vi "Read Needs rebuilding.vi"(11 "ProjectItem in":refnum<class "ProjectItem.lvclass">) -> (2 "Needs rebuilding":bool, 3 "ProjectItem out":refnum<class "ProjectItem.lvclass">)   [LabVIEW 2019, in "SolutionBuilder.lvlib" / "ProjectItem.lvclass"]
uses:
  ProjectItem.lvclass
  ProjectItem.lvclass/ProjectItem.ctl
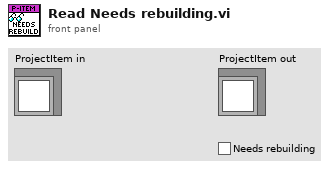
[diagram p1: front panel]
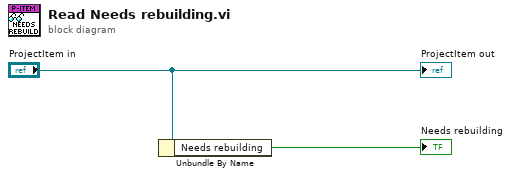
[diagram p0: block diagram]
diagram:
  n1 = Unbundle By Name("ProjectItem in") -> ("Needs rebuilding"=→"Needs rebuilding":bool)
  "ProjectItem out" <- "ProjectItem in"
